vi "Read remote port.vi"(8 "error in (no error)":errorcluster, 11 "Connection.TCP":refnum<class "Connection.TCP.lvclass">) -> (0 "error out":errorcluster, 2 "remote port":u16=80, 3 "Connection.TCP":refnum<class "Connection.TCP.lvclass">)   [LabVIEW 2013]
uses:
  <vilib>/LabVIEW Open Source Project/OpenURI/openURI.lvlib
  Connection.TCP.lvclass
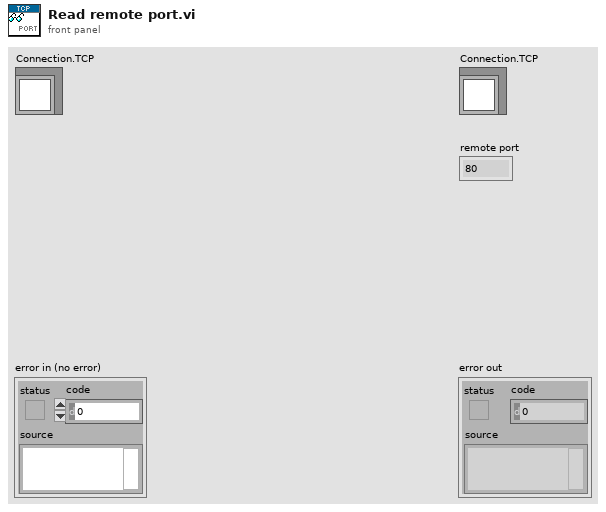
[diagram p1: front panel]
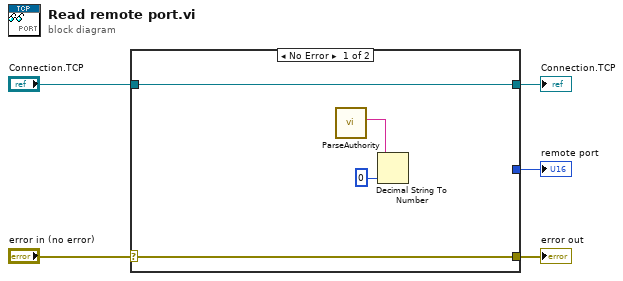
[diagram p0: block diagram]
diagram:
  n1 = case shown="No Error" "error in (no error)" {
    selector: "error in (no error)" -> [w9 w10]
    tunnel: [w9 w10] -> w4
    tunnel: [w8 w11] -> w2
    tunnel: "Connection.TCP" -> [w8 w11]
    tunnel: [_ _] -> w1
    frame No Error {
      n2 = call <vilib>:"ParseAuthority.vi"() -> ("port"=w7:string)  [unwired: 8 in, 3 out]
      n3 = Decimal String To Number(string=w7, default (0L)=u16 0 ("port")) -> ()  [unwired: 1 in, 2 out]
    }
    frame Error {
    }
  }
  "error out" <- w4
  "Connection.TCP" <- w2
  "remote port" <- w1
